vi "writeClusterWithDBReading.vi"(9 "datosClaseDB in":T1, 10 "readingData":string[](array[string]), 11 "tableName":string) -> (3 "datosClaseDB out":T1)   [LabVIEW 2014]
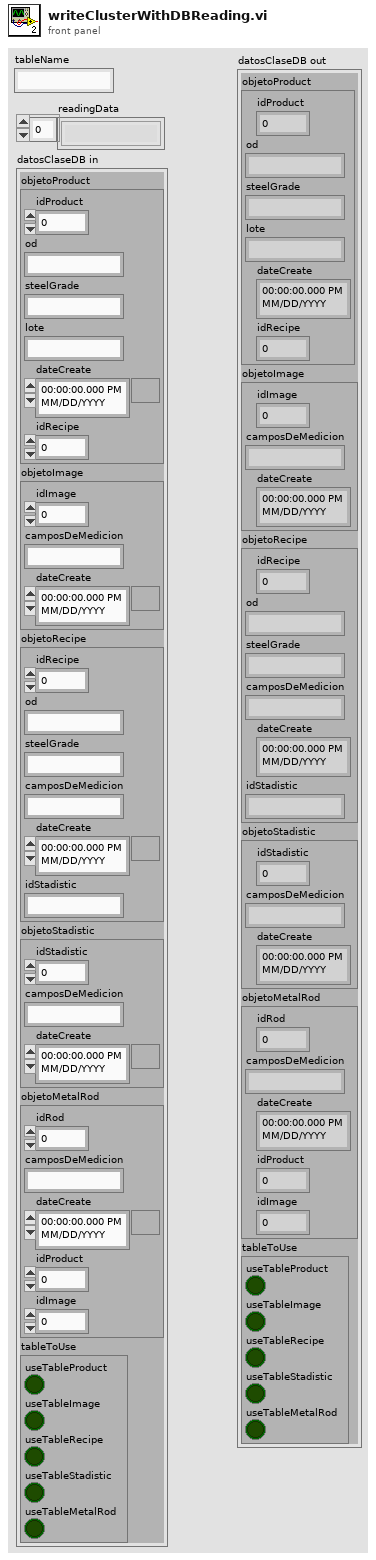
[diagram p1: front panel]
types:
  T1 = cluster{"objetoProduct":cluster{"idProduct":dbl, "od":string, "steelGrade":string, "lote":string, "dateCreate":timestamp, "idRecipe":dbl}, "objetoImage":cluster{"idImage":dbl, "camposDeMedicion":string, "dateCreate":timestamp}, "objetoRecipe":cluster{"idRecipe":dbl, "od":string, "steelGrade":string, "camposDeMedicion":string, "dateCreate":timestamp, "idStadistic":string}, "objetoStadistic":cluster{"idStadistic":dbl, "camposDeMedicion":string, "dateCreate":timestamp}, "objetoMetalRod":cluster{"idRod":dbl, "camposDeMedicion":string, "dateCreate":timestamp, "idProduct":dbl, "idImage":dbl}, "tableToUse":cluster{"useTableProduct":bool, "useTableImage":bool, "useTableRecipe":bool, "useTableStadistic":bool, "useTableMetalRod":bool}}
  T2 = cluster{"idProduct":dbl, "od":string, "steelGrade":string, "lote":string, "dateCreate":timestamp, "idRecipe":dbl}
  T3 = cluster{"idImage":dbl, "camposDeMedicion":string, "dateCreate":timestamp}
  T4 = cluster{"idRecipe":dbl, "od":string, "steelGrade":string, "camposDeMedicion":string, "dateCreate":timestamp, "idStadistic":string}
  T5 = cluster{"idStadistic":dbl, "camposDeMedicion":string, "dateCreate":timestamp}
  T6 = cluster{"idRod":dbl, "camposDeMedicion":string, "dateCreate":timestamp, "idProduct":dbl, "idImage":dbl}
  T7 = cluster{"useTableProduct":bool, "useTableImage":bool, "useTableRecipe":bool, "useTableStadistic":bool, "useTableMetalRod":bool}
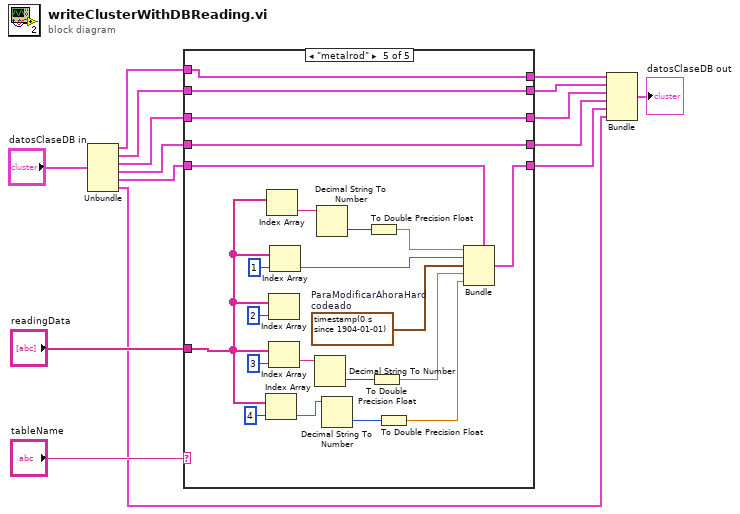
[diagram p0: block diagram]
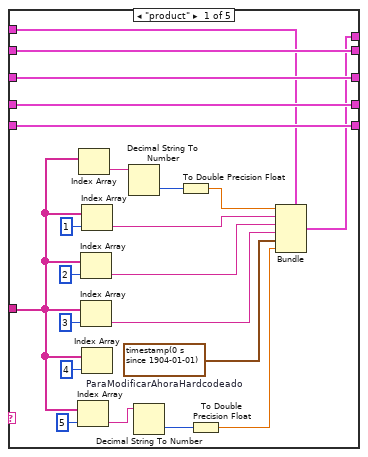
[diagram p2: hidden frame]
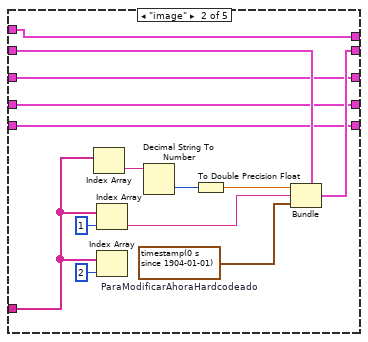
[diagram p3: hidden frame]
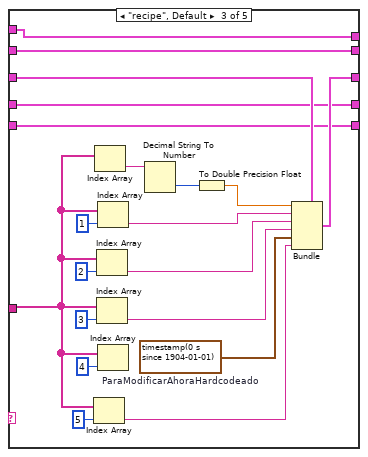
[diagram p4: hidden frame]
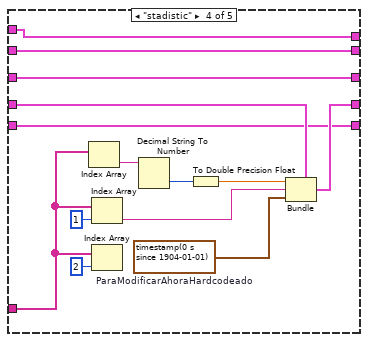
[diagram p5: hidden frame]
diagram:
  n1 = Unbundle("datosClaseDB in") -> ("objetoProduct"=w7:T2, "objetoImage"=w6:T3, "objetoRecipe"=w5:T4, "objetoStadistic"=w4:T5, "objetoMetalRod"=w3:T6, "tableToUse"=w2:T7)
  n2 = case shown="\"metalrod\"" "tableName" {
    tunnel: w7 -> [w16 w51 w71 w85 w107]
    tunnel: w6 -> [w37 w42 w70 w84 w106]
    tunnel: w5 -> [w36 w40 w55 w83 w105]
    tunnel: w4 -> [w35 w39 w53 w73 w104]
    tunnel: w3 -> [w34 w38 w52 w72 w92]
    tunnel: "readingData" -> [w28 w44 w57 w75 w93]
    tunnel: [w17 w51 w71 w85 w107] -> w13
    tunnel: [w37 w41 w70 w84 w106] -> w12
    tunnel: [w36 w40 w56 w83 w105] -> w11
    tunnel: [w35 w39 w53 w74 w104] -> w10
    tunnel: [w34 w38 w52 w72 w86] -> w9
    frame "product" {
      w20 = timestamp(0 s since 1904-01-01)  # ParaModificarAhoraHardcodeado
      n3 = Index Array(array=w28, index=5) -> (element=w26:string)
      n4 = Index Array(array=w28) -> (element=w33:string)  [unwired: 1 in]
      n5 = Index Array(array=w28, index=2) -> (element=w22:string)
      n6 = Index Array(array=w28, index=3) -> (element=w21:string)
      n7 = Index Array(array=w28, index=1) -> (element=w25:string)
      n8 = Index Array(array=w28, index=4) -> ()  [unwired: 1 out]
      n9 = Decimal String To Number(string=w33) -> (number=w24:i32)  [unwired: 2 in, 1 out]
      n10 = Decimal String To Number(string=w26) -> (number=w19:i32)  [unwired: 2 in, 1 out]
      n11 = To Double Precision Float(number=w24) -> (double precision float=w23:dbl)
      n12 = To Double Precision Float(number=w19) -> (double precision float=w18:dbl)
      n13 = Bundle(cluster=w16, "idProduct"=w23, "od"=w25, "steelGrade"=w22, "lote"=w21, "dateCreate"=w20, "idRecipe"=w18) -> (w17:T2)
    }
    frame "image" {
      w43 = timestamp(0 s since 1904-01-01)  # ParaModificarAhoraHardcodeado
      n14 = Index Array(array=w44) -> (element=w50:string)  [unwired: 1 in]
      n15 = Index Array(array=w44, index=1) -> (element=w47:string)
      n16 = Index Array(array=w44, index=2) -> ()  [unwired: 1 out]
      n17 = Decimal String To Number(string=w50) -> (number=w46:i32)  [unwired: 2 in, 1 out]
      n18 = To Double Precision Float(number=w46) -> (double precision float=w45:dbl)
      n19 = Bundle(cluster=w42, "idImage"=w45, "camposDeMedicion"=w47, "dateCreate"=w43) -> (w41:T3)
    }
    frame "recipe", Default {
      w58 = timestamp(0 s since 1904-01-01)  # ParaModificarAhoraHardcodeado
      n20 = Index Array(array=w57, index=5) -> (element=w54:string)
      n21 = Index Array(array=w57) -> (element=w69:string)  [unwired: 1 in]
      n22 = Index Array(array=w57, index=2) -> (element=w60:string)
      n23 = Index Array(array=w57, index=3) -> (element=w59:string)
      n24 = Index Array(array=w57, index=1) -> (element=w63:string)
      n25 = Index Array(array=w57, index=4) -> ()  [unwired: 1 out]
      n26 = Decimal String To Number(string=w69) -> (number=w62:i32)  [unwired: 2 in, 1 out]
      n27 = To Double Precision Float(number=w62) -> (double precision float=w61:dbl)
      n28 = Bundle(cluster=w55, "idRecipe"=w61, "od"=w63, "steelGrade"=w60, "camposDeMedicion"=w59, "dateCreate"=w58, "idStadistic"=w54) -> (w56:T4)
    }
    frame "stadistic" {
      w76 = timestamp(0 s since 1904-01-01)  # ParaModificarAhoraHardcodeado
      n29 = Index Array(array=w75) -> (element=w82:string)  [unwired: 1 in]
      n30 = Index Array(array=w75, index=1) -> (element=w79:string)
      n31 = Index Array(array=w75, index=2) -> ()  [unwired: 1 out]
      n32 = Decimal String To Number(string=w82) -> (number=w78:i32)  [unwired: 2 in, 1 out]
      n33 = To Double Precision Float(number=w78) -> (double precision float=w77:dbl)
      n34 = Bundle(cluster=w73, "idStadistic"=w77, "camposDeMedicion"=w79, "dateCreate"=w76) -> (w74:T5)
    }
    frame "metalrod" {
      w91 = timestamp(0 s since 1904-01-01)  # ParaModificarAhoraHardcodeado
      n35 = Index Array(array=w93, index=4) -> (element=w98:string)
      n36 = Index Array(array=w93) -> (element=w103:string)  [unwired: 1 in]
      n37 = Index Array(array=w93, index=2) -> ()  [unwired: 1 out]
      n38 = Index Array(array=w93, index=3) -> (element=w89:string)
      n39 = Index Array(array=w93, index=1) -> (element=w97:string)
      n40 = Decimal String To Number(string=w89) -> (number=w90:i32)  [unwired: 2 in, 1 out]
      n41 = Decimal String To Number(string=w103) -> (number=w96:i32)  [unwired: 2 in, 1 out]
      n42 = Decimal String To Number(string=w98) -> (number=w94:i32)  [unwired: 2 in, 1 out]
      n43 = To Double Precision Float(number=w96) -> (double precision float=w95:dbl)
      n44 = To Double Precision Float(number=w90) -> (double precision float=w88:dbl)
      n45 = To Double Precision Float(number=w94) -> (double precision float=w87:dbl)
      n46 = Bundle(cluster=w92, "idRod"=w95, "camposDeMedicion"=w97, "dateCreate"=w91, "idProduct"=w88, "idImage"=w87) -> (w86:T6)
    }
  }
  n47 = Bundle("objetoProduct"=w13, "objetoImage"=w12, "objetoRecipe"=w11, "objetoStadistic"=w10, "objetoMetalRod"=w9, "tableToUse"=w2) -> (→"datosClaseDB out":T1)  [unwired: 1 in]
